vi "gentec-SOLO_PE.Write.vi"(8 "error in (no error)":errorcluster, 9 "Parameters (Empty)":u32[](array[numeric]), 10 "Command Handle":u16, 11 "VISA Refnum in":refnum<visa-resource-name>) -> (0 "error out":errorcluster, 3 "VISA Refnum out":refnum<visa-resource-name>)   [LabVIEW 2014, in "gentec-SOLO-PE - Driver.lvlib"]
doc: "This VI calls a VISA Write."
uses:
  gentec-SOLO-PE - Driver.lvlib
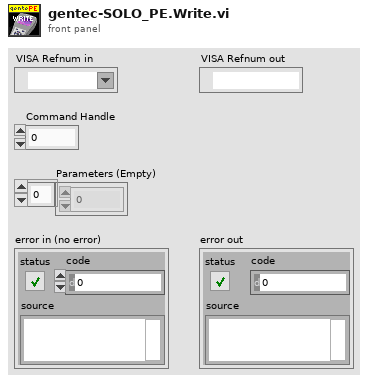
[diagram p1: front panel]
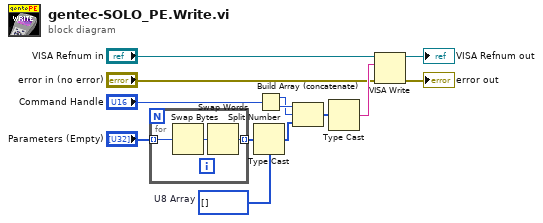
[diagram p0: block diagram]
diagram:
  w13 = u8[] []  # U8 Array
  n1 = for {
    tunnel: "Parameters (Empty)" -> [w15] mode=indexing
    tunnel: [w14] -> w5 mode=indexing
    n2 = Swap Bytes(anything=w15) -> (byte swapped=w16:u32)
    n3 = Swap Words(1:w16) -> (0:w14:u32)
  }
  n4 = Type Cast(type=w13, x=w5) -> (*(type *) &x=w1:u8[])
  n5 = Split Number(x="Command Handle") -> (hi(x)=w3:u8, lo(x)=w4:u8)
  n6 = Build Array (concatenate)(w4, w3, w1) -> (w2:u8[])
  n7 = Type Cast(x=w2) -> (*(type *) &x=w12:string)  [unwired: 1 in]
  n8 = VISA Write(VISA resource name="VISA Refnum in", write buffer=w12, error in (no error)="error in (no error)") -> (VISA resource name out=→"VISA Refnum out":refnum<visa-resource-name>, error out=→"error out":errorcluster)  [unwired: 1 out]
